vi "LSX Get EEP Rom Value.vi"(8 "error in (no error)":errorcluster, 9 "pValue":string, 10 "Offset":u8, 11 "lLSID":i32) -> (0 "error out":errorcluster, 1 "pValue out":string, 3 "function return":i32)   [LabVIEW 2016, in "Tango_DLL.lvlib"]
doc: "TANGOAPI int TANGOCALL LSX_GetEEPRomValue (int lLSID, byte Offset, byte *pValue);"
uses:
  Tango_DLL.lvlib
  2017/Microscope Control/Device Library/Stages/Marzhauser/SCAN IM 120 x 80/Tango DLL VIs/Tango_DLL.dll
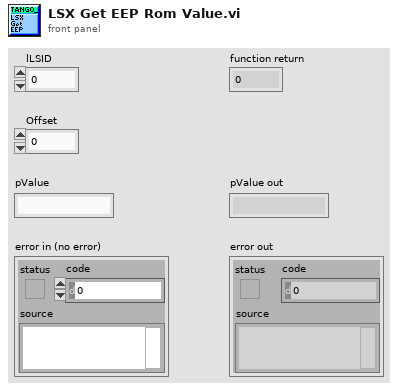
[diagram p1: front panel]
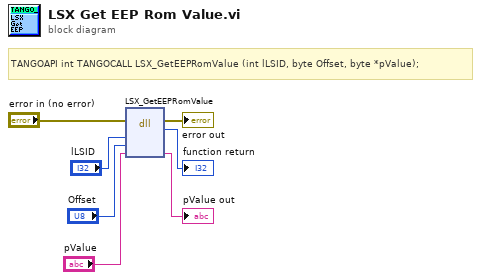
[diagram p0: block diagram]
diagram:
  # "TANGOAPI int TANGOCALL LSX_GetEEPRomValue (int lLSID, byte Offset, byte *pValue);"
  n1 = dll-call lib="C:/Users/4PiSMS/Documents/Microscope Control/2017/Microscope Control/Device Library/Stages/Marzhauser/SCAN IM 120 x 80/Tango DLL VIs/Tango_DLL.*" fn="LSX_GetEEPRomValue"(error in="error in (no error)", "lLSID"="lLSID", "Offset"="Offset", "pValue"="pValue") -> (error out=→"error out":errorcluster, →"function return":i32, "pValue"=→"pValue out":string)  [unwired: 4 in, 1 out]
